vi "table_test.vi"() -> ()   [LabVIEW 2019]
panel:
  out "Table":string[][](table)
  out "String 2":string
  out "String":string
  in  "stop":bool
  in  "OK Button":bool
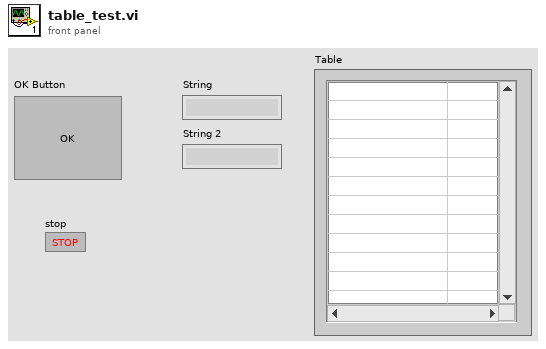
[diagram p1: front panel]
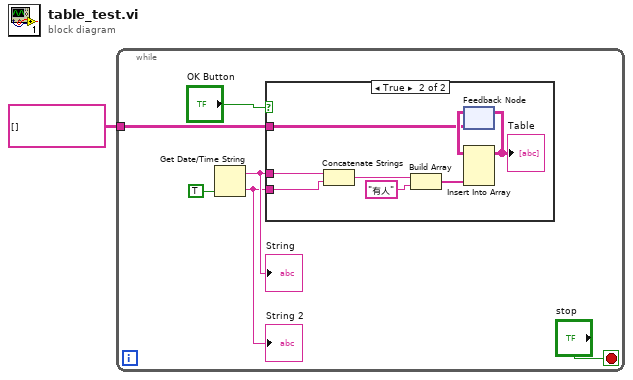
[diagram p0: block diagram]
diagram:
  n1 = while {
    tunnel: string[][] [] -> [w2]
    stop <- "stop" stop-if-true
    n2 = Get Date/Time String(want seconds? (F)=TRUE) -> (date string=w5:string, time string=w4:string)  [unwired: 2 in]
    "String" <- w5
    "String 2" <- w4
    n3 = case shown="True" "OK Button" {
      tunnel: w5 -> [_ w15]
      tunnel: w4 -> [_ w14]
      tunnel: w2 -> [_ w9]
      frame False {
      }
      frame True {
        n4 = Concatenate Strings(w15, w14) -> (w12:string)
        n5 = Build Array(w12, "有人") -> (w11:string[])
        n6 = feedback #1(w9) -> (w10:string[][])
        n7 = Insert Into Array(array=w10, new element=w11) -> (w8:string[][])  [unwired: 2 in]
        "Table" <- w8
        n8 = feedback-in #1(w8) -> ()
      }
    }
  }
